vi "extract pv info.vi"(8 "error in":errorcluster, 10 "PV Info":T1[](array[typedef]), 11 "CA in":T2) -> (0 "error out":errorcluster, 2 "PV Selected":T1)   [LabVIEW 2022 SP3]
uses:
  Program Files/National Instruments/LabVIEW 2023/user.lib/calab/PV Info.ctl
  Program Files/National Instruments/LabVIEW 2023/user.lib/calab/CaLab.lvlib
  pectus/control/ca cluster.ctl
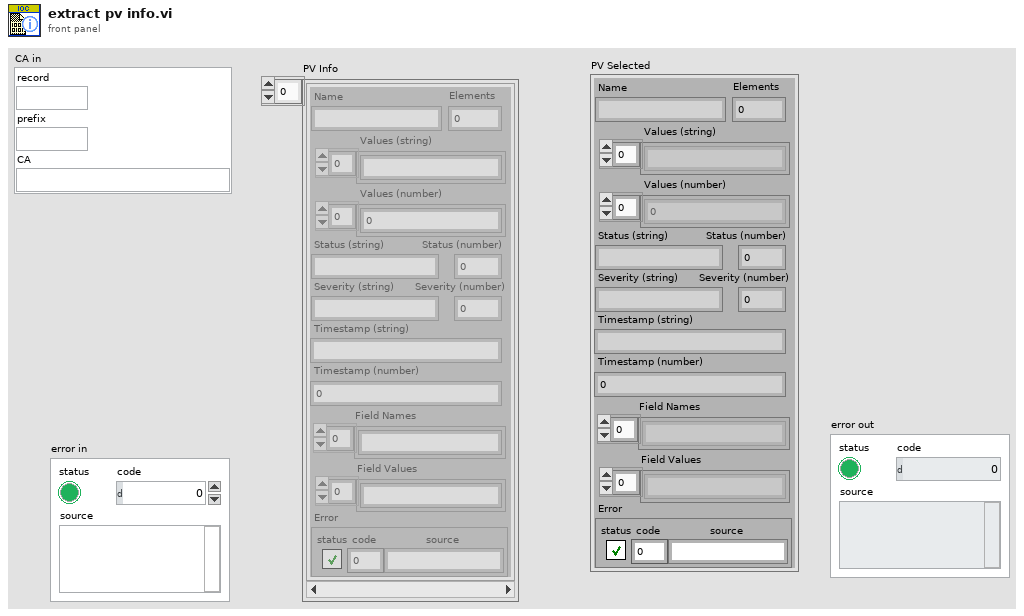
[diagram p1: front panel]
types:
  T1 = typedef "CaLab.lvlib/PV Info.ctl" = cluster{"Name":string, "Elements":i32, "Values (string)":string[], "Values (number)":dbl[], "Status (string)":string, "Status (number)":i16, "Severity (string)":string, "Severity (number)":i16, "Timestamp (string)":string, "Timestamp (number)":i32, "Field Names":string[], "Field Values":string[], "Error":errorcluster}
  T2 = typedef "ca cluster.ctl" = cluster{"record":string, "prefix":string, "CA":string}
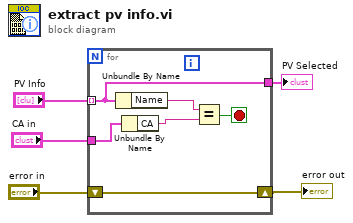
[diagram p0: block diagram]
diagram:
  n1 = for {
    tunnel: "PV Info" -> [w10] mode=indexing
    tunnel: "CA in" -> [w7]
    tunnel: [w10] -> w1
    shift-right: [w9] -> w2
    shift-left: "error in" -> [w9]
    stop <- w8 stop-if-true
    n2 = Unbundle By Name(w10) -> ("Name"=w11:string)
    n3 = Unbundle By Name(w7) -> ("CA"=w6:string)
    n4 = Equal?(x=w11, y=w6) -> (x = y?=w8:bool)
  }
  "error out" <- w2
  "PV Selected" <- w1
